vi "Error_Control.vi"(0 "ERD Loop":refnum<queue>, 1 "GEA2":refnum<queue>, 2 "Command (Handle Errors)":T1=enum."Handle Errors", 5 "Receive Loop":refnum<user-event>, 7 "UI Loop Error":refnum<user-event>, 11 "Error In":errorcluster) -> (15 "Error Out":errorcluster)   [LabVIEW 2023]
uses:
  type defs/Error_Command.ctl
  type defs/ERD_Data_Loop_Control.ctl
  type defs/ERD_Loop_States.ctl
  GExplorer Support/typedefs/GExplorer_Data_Cluster.ctl
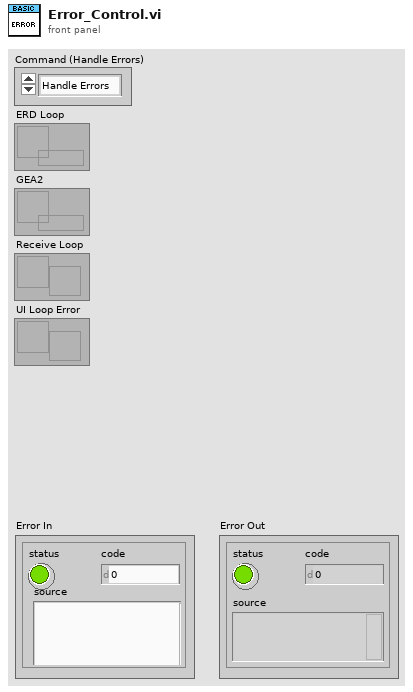
[diagram p1: front panel]
types:
  T1 = typedef "Error_Command.ctl" = enum16{"Initialize", "Handle Errors", "Report Errors"}
  T2 = typedef "ERD_Data_Loop_Control.ctl" = cluster{"Data":variant, "State":T3}
  T3 = typedef "ERD_Loop_States.ctl" = enum16{"Init", "Build ERD Read List", "Read ERDs", "Get Version", "ERD´s User show", "Update UI", "Graph", "Read Faults", "Log Data", "Pause", "Shutdown"}
  T4 = typedef "GExplorer_Data_Cluster.ctl" = cluster{"Data":variant, "State":enum16{"Add to Log", "Clear", "Shutdown"}}
  T5 = typedef "Ref_ReceiveLoop_UserEvent.ctl" = refnum<user-event>
  T6 = typedef "Ref_UILoop_UserEvent.ctl" = refnum<user-event>
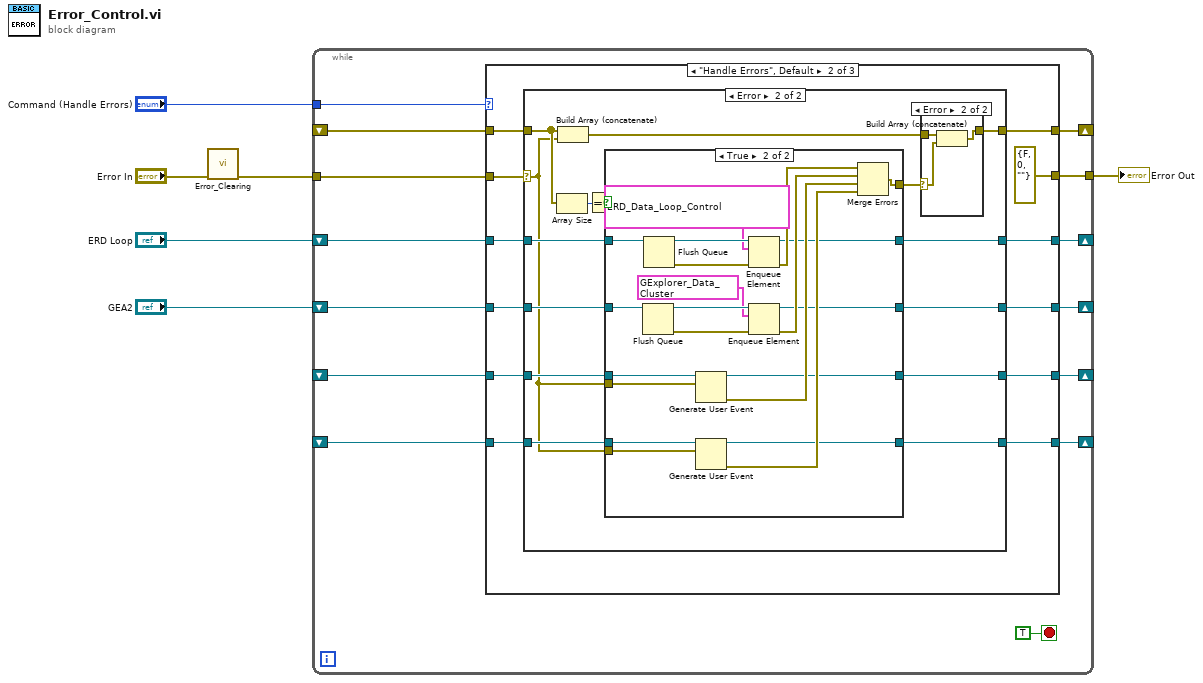
[diagram p0: block diagram]
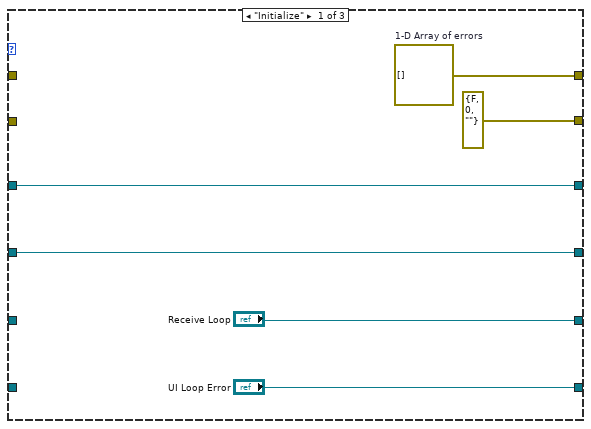
[diagram p2: hidden frame]
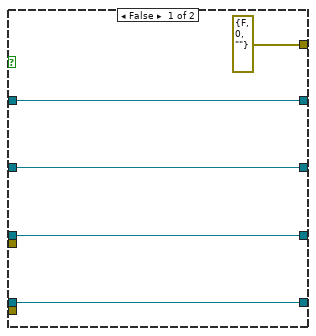
[diagram p4: hidden frame]
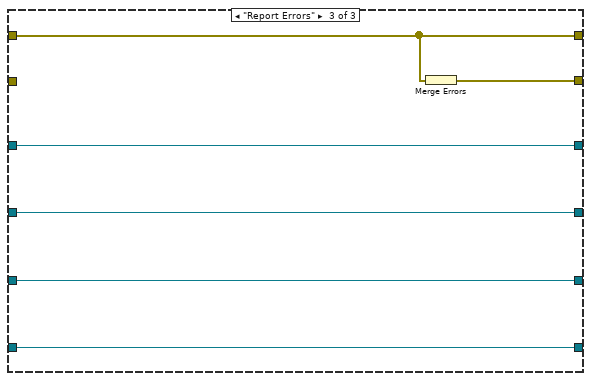
[diagram p6: hidden frame]
diagram:
  n1 = call "Error_Clearing.vi"("error in (no error)"="Error In") -> ("error out"=w1:errorcluster)  [unwired: 10 in]
  n2 = while {
    tunnel: w1 -> [w18]
    tunnel: "Command (Handle Errors)" -> [w19]
    shift-right: [w17] -> _
    shift-left: _ -> [w16]
    tunnel: [w15] -> w4
    shift-right: [w14] -> _
    shift-left: "ERD Loop" -> [w10]
    shift-right: [w13] -> _
    shift-left: "GEA2" -> [w9]
    shift-right: [w12] -> _
    shift-left: _ -> [w8]
    shift-right: [w11] -> _
    shift-left: _ -> [w7]
    stop <- TRUE stop-if-true
    n3 = case shown="\"Handle Errors\", Default" w19 {
      tunnel: w18 -> [_ w38 _]
      tunnel: [w26 w32 w93] -> w17
      tunnel: w16 -> [_ w37 w93]
      tunnel: [errorcluster {"status"=FALSE, "code"=0, "source"=""} ("Error In") errorcluster {"status"=FALSE, "code"=0, "source"=""} ("Error In") w94] -> w15
      tunnel: [w24 w30 w92] -> w14
      tunnel: [w23 w31 w91] -> w13
      tunnel: ["Receive Loop" w29 w90] -> w12
      tunnel: ["UI Loop Error" w28 w89] -> w11
      tunnel: w10 -> [w24 w36 w92]
      tunnel: w9 -> [w23 w35 w91]
      tunnel: w8 -> [_ w34 w90]
      tunnel: w7 -> [_ w33 w89]
      frame "Initialize" {
        w26 = errorcluster[] []  # 1-D Array of errors
      }
      frame "Handle Errors", Default {
        n4 = case shown="Error" w38 {
          selector: w38 -> [_ w49]
          tunnel: w37 -> [w43 w58]
          tunnel: w36 -> [w42 w55]
          tunnel: w35 -> [w41 w54]
          tunnel: w34 -> [w40 w53]
          tunnel: w33 -> [w39 w52]
          tunnel: [w43 w50] -> w32
          tunnel: [w41 w48] -> w31
          tunnel: [w42 w47] -> w30
          tunnel: [w40 w46] -> w29
          tunnel: [w39 w45] -> w28
          frame No Error {
          }
          frame Error {
            n5 = Array Size(array=w58) -> (size(s)=w57:i32)
            n6 = Build Array (concatenate)(w58, w49) -> (w44:errorcluster[])
            n7 = Equal To 0?(x=w57) -> (x = 0?=w56:bool)
            n8 = case shown="True" w56 {
              tunnel: w55 -> [w62 w84]
              tunnel: w54 -> [w61 w83]
              tunnel: w53 -> [w60 w75]
              tunnel: w52 -> [w59 w73]
              tunnel: [errorcluster {"status"=FALSE, "code"=0, "source"=""} ("error IO") w82] -> w51
              tunnel: w49 -> [_ w74]
              tunnel: w49 -> [_ w72]
              tunnel: [w61 w67] -> w48
              tunnel: [w62 w66] -> w47
              tunnel: [w60 w65] -> w46
              tunnel: [w59 w64] -> w45
              frame False {
              }
              frame True {
                n9 = Flush Queue(queue=w83) -> (queue out=w80:refnum<queue>, error out=w81:errorcluster)  [unwired: 1 in, 1 out]
                n10 = Flush Queue(queue=w84) -> (queue out=w77:refnum<queue>, error out=w78:errorcluster)  [unwired: 1 in, 1 out]
                n11 = Generate User Event(user event=w75, event data cluster=w74) -> (user event out=w65:T5, error out=w70:errorcluster)  [unwired: 2 in]
                n12 = Generate User Event(user event=w73, event data cluster=w72) -> (user event out=w64:T6, error out=w71:errorcluster)  [unwired: 2 in]
                n13 = Enqueue Element(queue=w77, element=T2 {"Data"=variant, "State"=enum."Shutdown"}, error in (no error)=w78) -> (queue out=w66:refnum<queue>, error out=w69:errorcluster)  [unwired: 1 in, 1 out]
                n14 = Enqueue Element(queue=w80, element=T4 {"Data"=variant, "State"=enum."Shutdown"}, error in (no error)=w81) -> (queue out=w67:refnum<queue>, error out=w68:errorcluster)  [unwired: 1 in, 1 out]
                n15 = Merge Errors(w69, w68, w70, w71) -> (w82:errorcluster)
              }
            }
            n16 = case shown="Error" w51 {
              selector: w51 -> [_ w87]
              tunnel: [w85 w88] -> w50
              tunnel: w44 -> [w85 w86]
              frame No Error {
              }
              frame Error {
                n17 = Build Array (concatenate)(w86, w87) -> (w88:errorcluster[])
              }
            }
          }
        }
      }
      frame "Report Errors" {
        n18 = Merge Errors(w93) -> (w94:errorcluster)
      }
    }
  }
  "Error Out" <- w4
